vi "Start Chassis.vi"(5 "Cfg wChassis":T1, 6 "Show FP?":bool, 7 "Actor-to-Caller Enqueuer":refnum<class "Message Enqueuer.lvclass">, 8 "error in (no error)":errorcluster, 9 "TCP LS Writer":refnum<class "Message Enqueuer.lvclass">, 10 "TCP HS Writer":refnum<class "Message Enqueuer.lvclass">, 11 "LS Only in":refnum<class "LS Only.lvclass">) -> (0 "error out":errorcluster, 3 "LS Only out":refnum<class "LS Only.lvclass">)   [LabVIEW 2012, in "Data Acquisition.lvlib" / "LS Only.lvclass"]
uses:
  LS Only.lvclass
  <vilib>/ActorFramework/Message Enqueuer/Message Enqueuer.lvclass
  Custom Ctrls/Master Cfg/ge_Cfg wChassis.ctl
  Cfg Grandmaster/Class Chassis BOM/Chassis BOM.lvclass
  Cfg Grandmaster/Class Chassis Cfg/ChassisCfg.lvclass
  Class Chassis Tasks/Chassis Tasks.lvclass
  Common/Controls/TE_Designator.ctl
  Class DAQ Actor/DAQ Actor.lvclass
  Class Chassis Tasks/Chassis Tasks.lvclass/Chassis Tasks.ctl
  <vilib>/ActorFramework/Message Enqueuer/Message Enqueuer.lvclass/Message Enqueuer.ctl
  Class Chassis Tasks/Read LS DAQ Task.vi
  Class Chassis Tasks/Write LS ActorQ.vi
  <vilib>/ActorFramework/Message Enqueuer/Enqueue.vi
  <vilib>/ActorFramework/Message Priority Queue/Priority Enqueue.vi
  Class DAQ Task/DAQ Task.lvclass
  DAQ Actor Messages/Start Task Msg/Start Task Msg.lvclass
  <vilib>/ActorFramework/Actor/Actor.lvclass
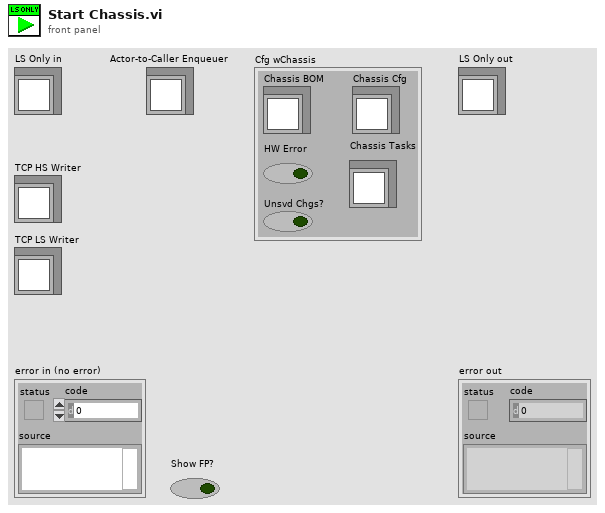
[diagram p1: front panel]
types:
  T1 = typedef "ge_Cfg wChassis.ctl" = cluster{"Chassis BOM":refnum<class "Chassis BOM.lvclass">, "Chassis Cfg":refnum<class "ChassisCfg.lvclass">, "Chassis Tasks":refnum<class "Chassis Tasks.lvclass">, "HW Error":bool, "Unsvd Chgs?":bool}
  T2 = typedef "TE_Designator.ctl" = enum16{"High Speed", "Low Speed"}
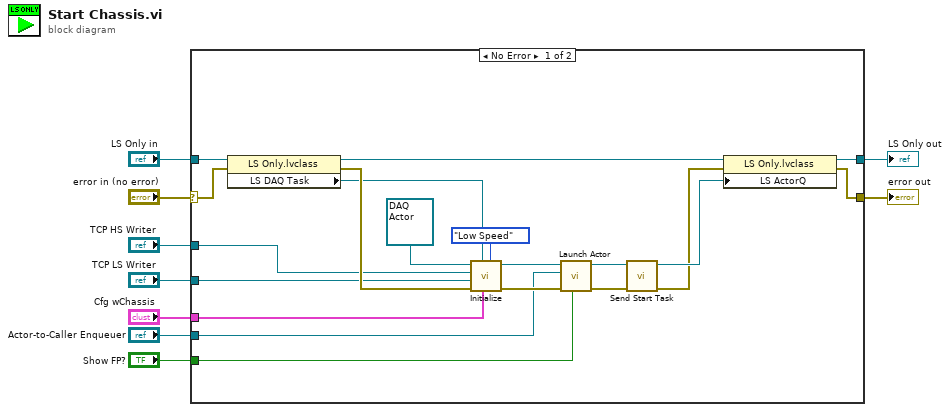
[diagram p0: block diagram]
diagram:
  n1 = case shown="No Error" "error in (no error)" {
    selector: "error in (no error)" -> [w14 w31]
    tunnel: "Actor-to-Caller Enqueuer" -> [w24 _]
    tunnel: "Cfg wChassis" -> [w12 _]
    tunnel: "LS Only in" -> [w23 w30]
    tunnel: [w20 w30] -> w6
    tunnel: [w19 w31] -> w5
    tunnel: "TCP LS Writer" -> [w18 _]
    tunnel: "TCP HS Writer" -> [w17 _]
    tunnel: "Show FP?" -> [w10 _]
    frame No Error {
      n2 = property class="LS Only.lvclass"(reference=w23, error in=w14) -> (reference out=w21:refnum<class "LS Only.lvclass">, error out=w22:errorcluster, "LS DAQ Task"=w13:refnum<class "DAQ Task.lvclass">)
      n3 = call-dynamic "Initialize.vi"("TimingEngine"=TE_Designator."Low Speed", "Cfg wChassis"=w12, "LS DAQ Task"=w13, "error in (no error)"=w22, "TCP LS Writer"=w18, "TCP HS Writer"=w17, "DAQ Actor in"=refnum<class "DAQ Actor.lvclass"> refnum) -> ("error out"=w29:errorcluster, "DAQ Actor out"=w28:refnum<class "DAQ Actor.lvclass">)  [unwired: 3 in]
      n4 = call <vilib>:"Launch Actor.vi"("Open Actor Core front panel? (F)"=w10, "error in (no error)"=w29, "Actor-to-Caller Enqueuer"=w24, "Actor"=w28) -> ("error out"=w25:errorcluster, "Caller-To-Actor Enqueuer"=w26:refnum<class "Message Enqueuer.lvclass">)  [unwired: 6 in]
      n5 = call "Send Start Task.vi"("error in (no error)"=w25, "Message Enqueuer"=w26) -> ("error out"=w15:errorcluster, "Message Enqueuer out"=w16:refnum<class "Message Enqueuer.lvclass">)  [unwired: 8 in]
      n6 = property class="LS Only.lvclass"(reference=w21, error in=w15, "LS ActorQ"=w16) -> (reference out=w20:refnum<class "LS Only.lvclass">, error out=w19:errorcluster)
    }
    frame Error {
    }
  }
  "error out" <- w5
  "LS Only out" <- w6
